vi "MsgProcessError.vi"() -> (1 "message name":string)   [LabVIEW 2017, in "Qbus.lvclass"]
uses:
  <vilib>/addons/Qbus/Qbus.lvclass
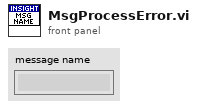
[diagram p1: front panel]
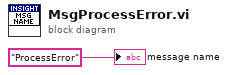
[diagram p0: block diagram]
diagram:
  "message name" <- "ProcessError" ("Qprocess")
